vi "Dual Signal FFT.vi"(0 "Signal 1":dbl[](array[numeric]) format="%.2f", 1 "Signal 2":dbl[](array[numeric]) format="%.2f") -> (2 "FFT 1":cdb[](array[numeric]) format="%.2f", 3 "FFT 2":cdb[](array[numeric]) format="%.2f", 4 "error":i32)   [LabVIEW 2018, in "NI_Gmath.lvlib"]
doc: "One step computation of the Fourier transforms of two real signals of equal length."
uses:
  NI_Gmath.lvlib
  Complex FFT.vi
  <vilib>/Analysis/NI_AALPro.lvlib
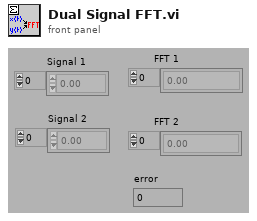
[diagram p1: front panel]
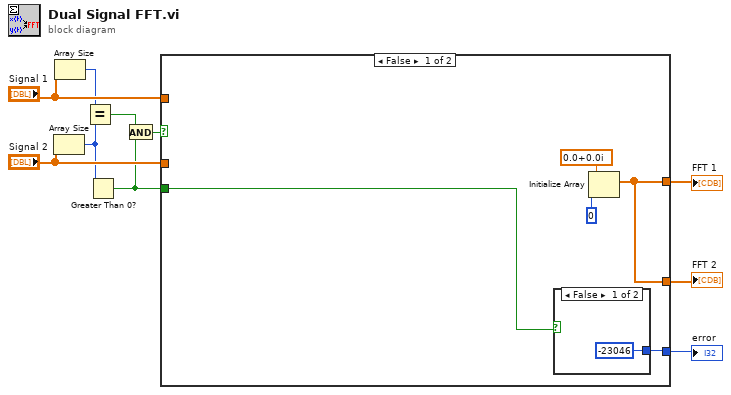
[diagram p0: block diagram]
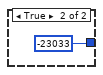
[diagram p2: hidden frame]
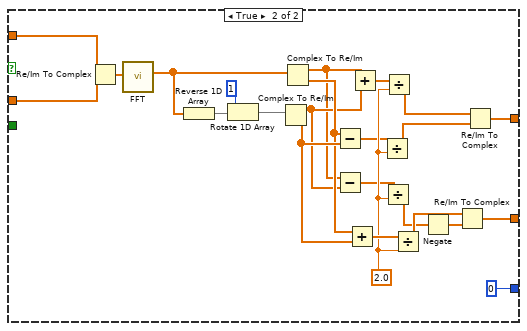
[diagram p3: hidden frame]
diagram:
  n1 = Array Size(array="Signal 2") -> (size(s)=w3:i32)
  n2 = Array Size(array="Signal 1") -> (size(s)=w5:i32)
  n3 = Equal?(x=w5, y=w3) -> (x = y?=w4:bool)
  n4 = Greater Than 0?(x=w3) -> (x > 0?=w1:bool)
  n5 = And(x=w4, y=w1) -> (x .and. y?=w2:bool)
  n6 = case shown="False" w2 {
    tunnel: "Signal 2" -> [_ w41]
    tunnel: "Signal 1" -> [_ w33]
    tunnel: [w13 w28] -> w9
    tunnel: [w13 w24] -> w10
    tunnel: [w11 0] -> w8
    tunnel: w1 -> [w12 _]
    frame False {
      n7 = case shown="False" w12 {
        tunnel: [-23046 -23033] -> w11
        frame False {
        }
        frame True {
        }
      }
      n8 = Initialize Array(cdb 0.0+0.0i, 0) -> (w13:cdb[])
    }
    frame True {
      w29 = 2.0
      n9 = Re/Im To Complex(1:w41, 2:w33) -> (0:w19:cdb[])
      n10 = call-poly "FFT.vi"("X"=w19) -> ("FFT {X}"=w20:cdb[])  [unwired: 9 in, 1 out]
      n11 = Reverse 1D Array(array=w20) -> (reversed array=w35:cdb[])
      n12 = Rotate 1D Array(1:w35, 2:1) -> (0:w37:cdb[])
      n13 = Complex To Re/Im(x + iy=w37) -> (x=w26:dbl[], y=w31:dbl[])
      n14 = Complex To Re/Im(x + iy=w20) -> (x=w25:dbl[], y=w30:dbl[])
      n15 = Subtract(x=w30, y=w31) -> (x-y=w22:dbl[])
      n16 = Subtract(x=w25, y=w26) -> (x-y=w27:dbl[])
      n17 = Add(x=w30, y=w31) -> (x+y=w32:dbl[])
      n18 = Add(x=w25, y=w26) -> (x+y=w21:dbl[])
      n19 = Divide(x=w22, y=w29) -> (x/y=w34:dbl[])
      n20 = Divide(x=w27, y=w29) -> (x/y=w38:dbl[])
      n21 = Divide(x=w21, y=w29) -> (x/y=w23:dbl[])
      n22 = Divide(x=w32, y=w29) -> (x/y=w40:dbl[])
      n23 = Negate(x=w38) -> (-x=w39:dbl[])
      n24 = Re/Im To Complex(1:w39, 2:w40) -> (0:w28:cdb[])
      n25 = Re/Im To Complex(1:w34, 2:w23) -> (0:w24:cdb[])
    }
  }
  "FFT 1" <- w10
  "FFT 2" <- w9
  "error" <- w8
